vi "WriteData.vi"(6 "TransmissionType":T1, 8 "error in (no error)":errorcluster, 10 "Command":string, 11 "ControlState in":T2 {"ChainMask" format="0x%02x"}) -> (0 "error out":errorcluster, 1 "Data Written?":bool, 2 "return count":u32, 3 "ControlState out":T2 {"ChainMask" format="0x%02x"})   [LabVIEW 2018, in "ArduinoSerialBling.lvlib"]
uses:
  ArduinoSerialBling.lvlib
  ControlState.ctl
  ConnectionType.ctl
  UdpConnection.ctl
  ChainState.ctl
  TransmissionType.ctl
  <vilib>/Instr/_visa.llb/VISA Flush IO Buffer Mask.ctl
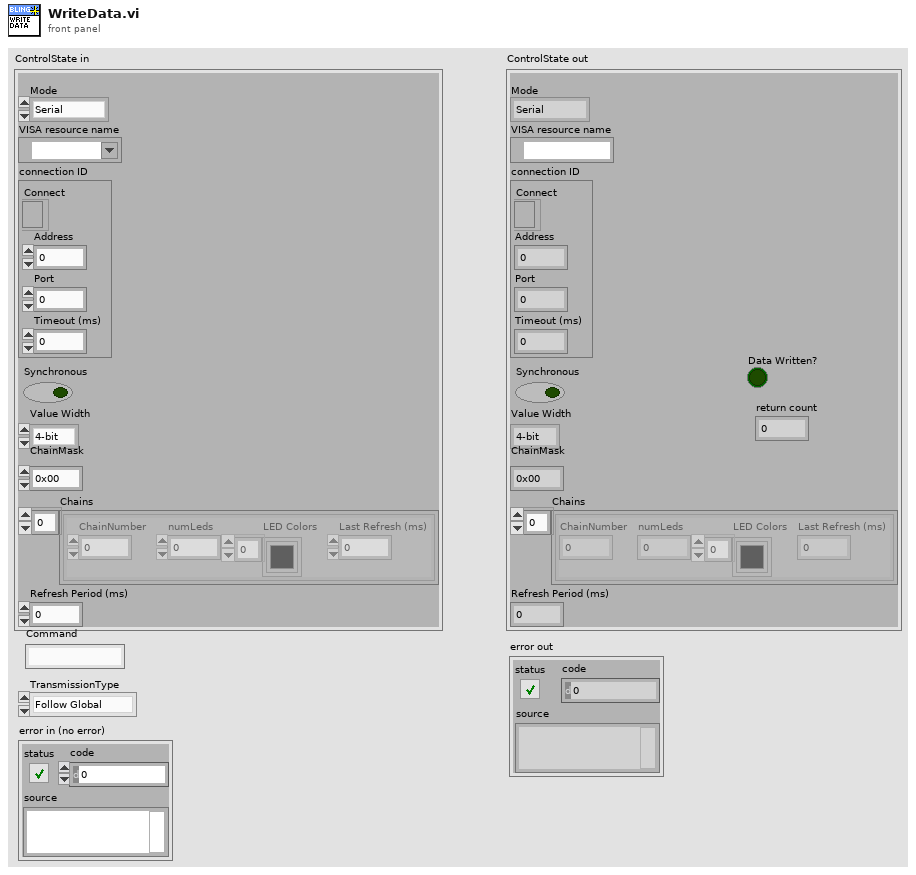
[diagram p1: front panel]
types:
  T1 = typedef "ArduinoSerialBling.lvlib/TransmissionType.ctl" = enum16{"Follow Global", "Asynchronous", "Synchronous"}
  T2 = typedef "ArduinoSerialBling.lvlib/ControlState.ctl" = cluster{"Mode":T3, "VISA resource name":refnum<visa-resource-name>, "connection ID":T4, "Synchronous":bool, "Value Width":enum16{"4-bit", "8-bit"}, "ChainMask":u8, "Chains":T5[], "Refresh Period (ms)":u32}
  T3 = typedef "ConnectionType.ctl" = enum16{"Serial", "Ethernet", "Offline"}
  T4 = typedef "UdpConnection.ctl" = cluster{"Connect":refnum<k16>, "Address":u32, "Port":u16, "Timeout (ms)":i32}
  T5 = typedef "ArduinoSerialBling.lvlib/ChainState.ctl" = cluster{"ChainNumber":u8, "numLeds":u8, "LED Colors":u32[], "Last Refresh (ms)":u32}
  T6 = typedef "VISA Flush IO Buffer Mask.ctl" = u16
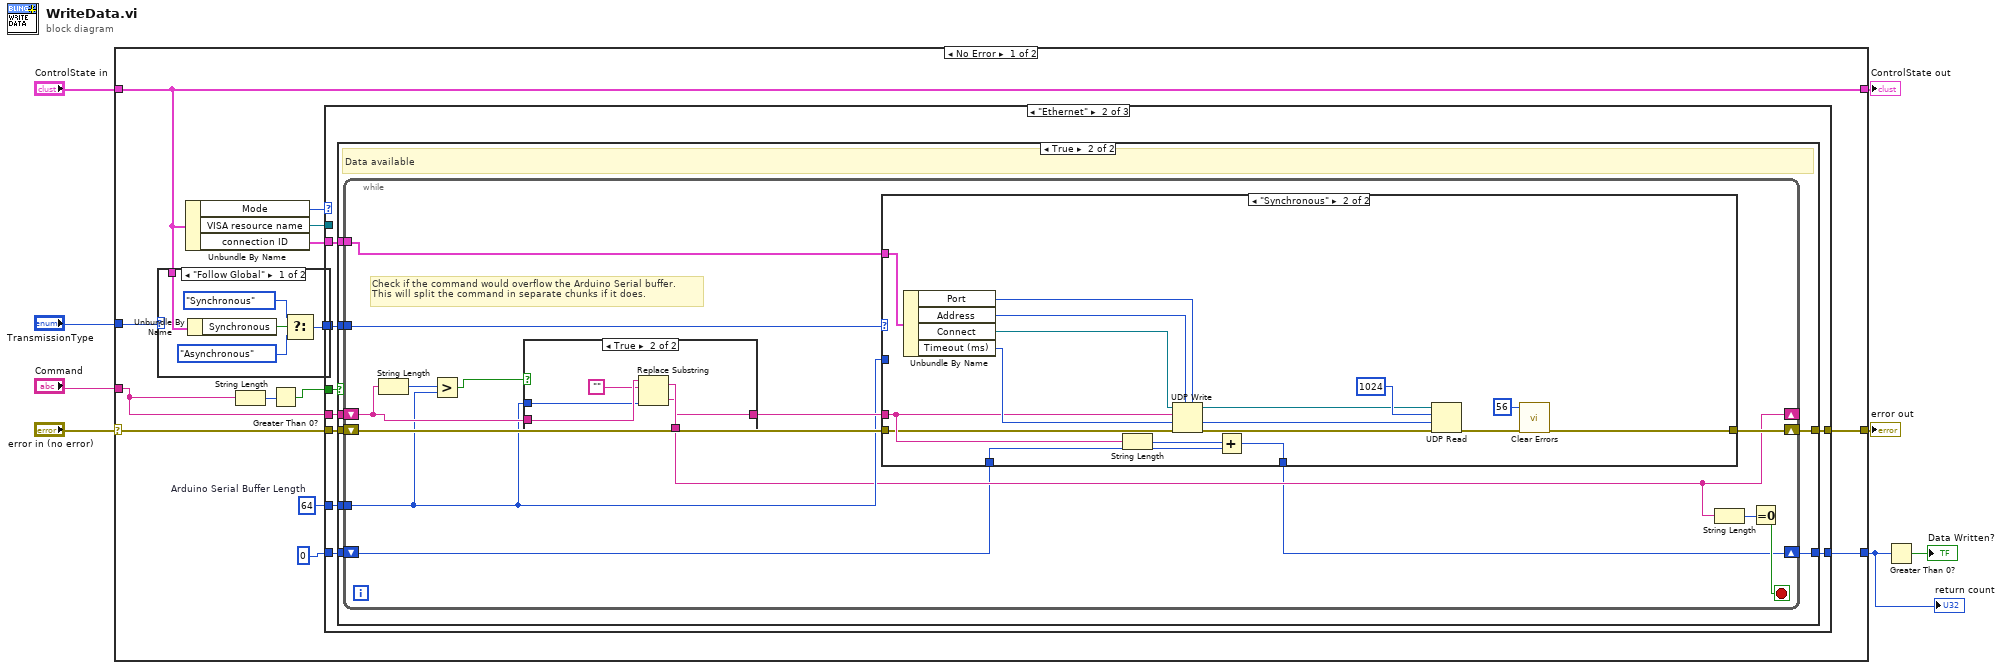
[diagram p0: block diagram]
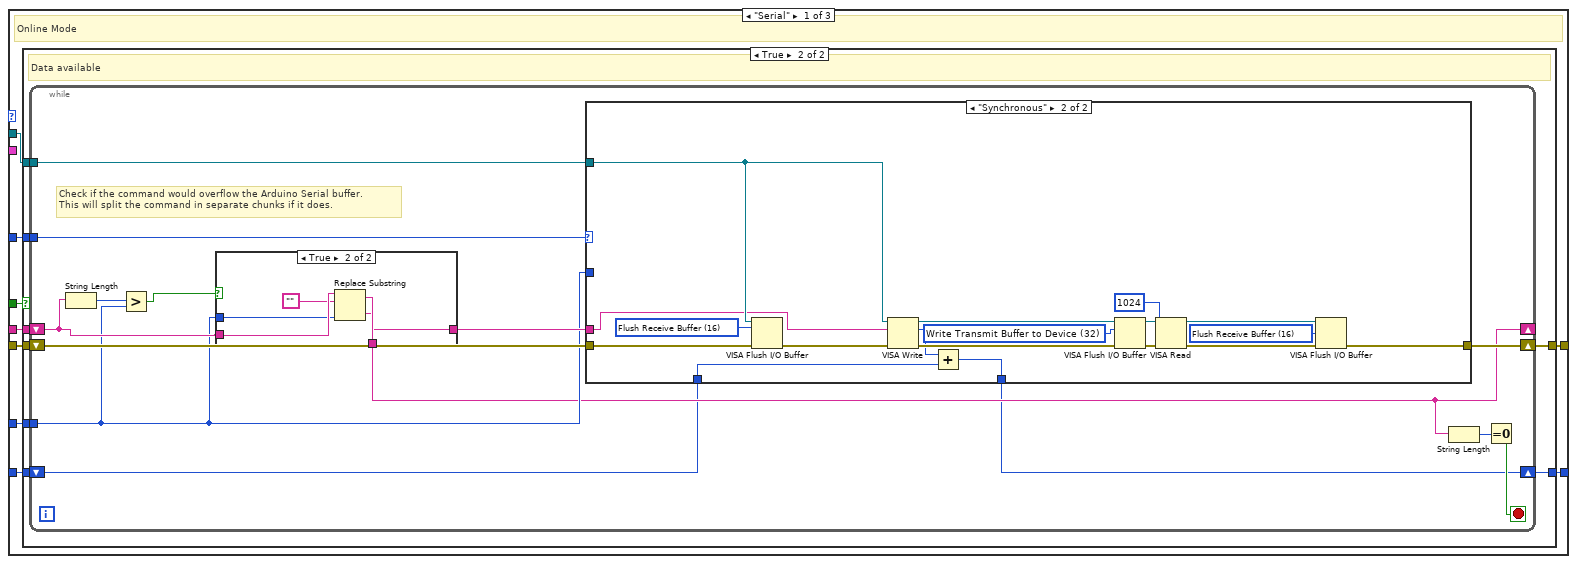
[diagram p2: hidden frame]
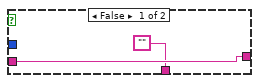
[diagram p4: hidden frame]
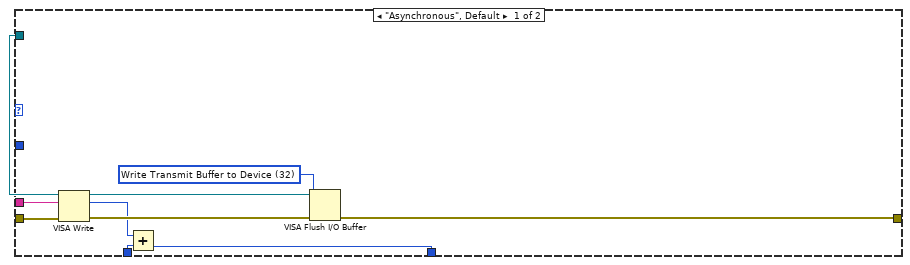
[diagram p5: hidden frame]
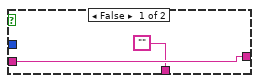
[diagram p7: hidden frame]
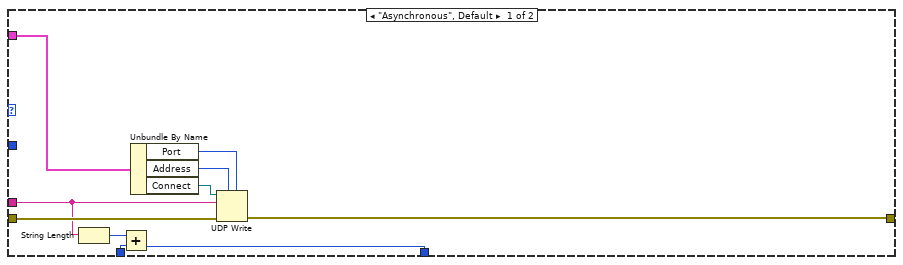
[diagram p8: hidden frame]
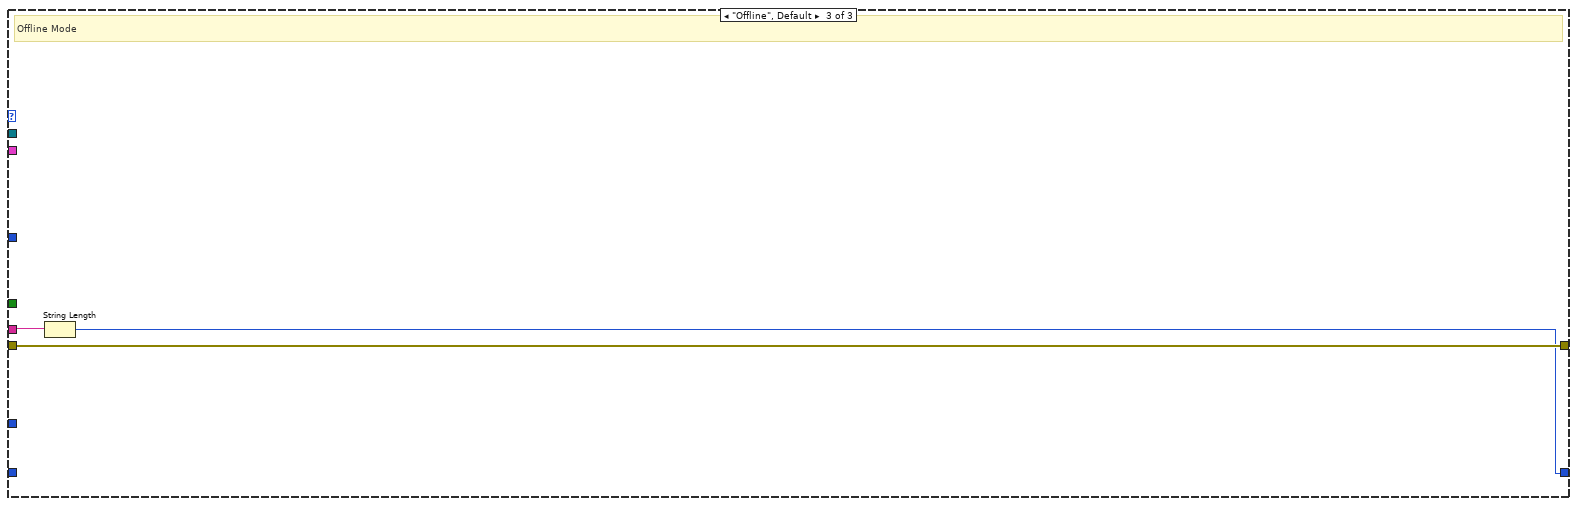
[diagram p9: hidden frame]
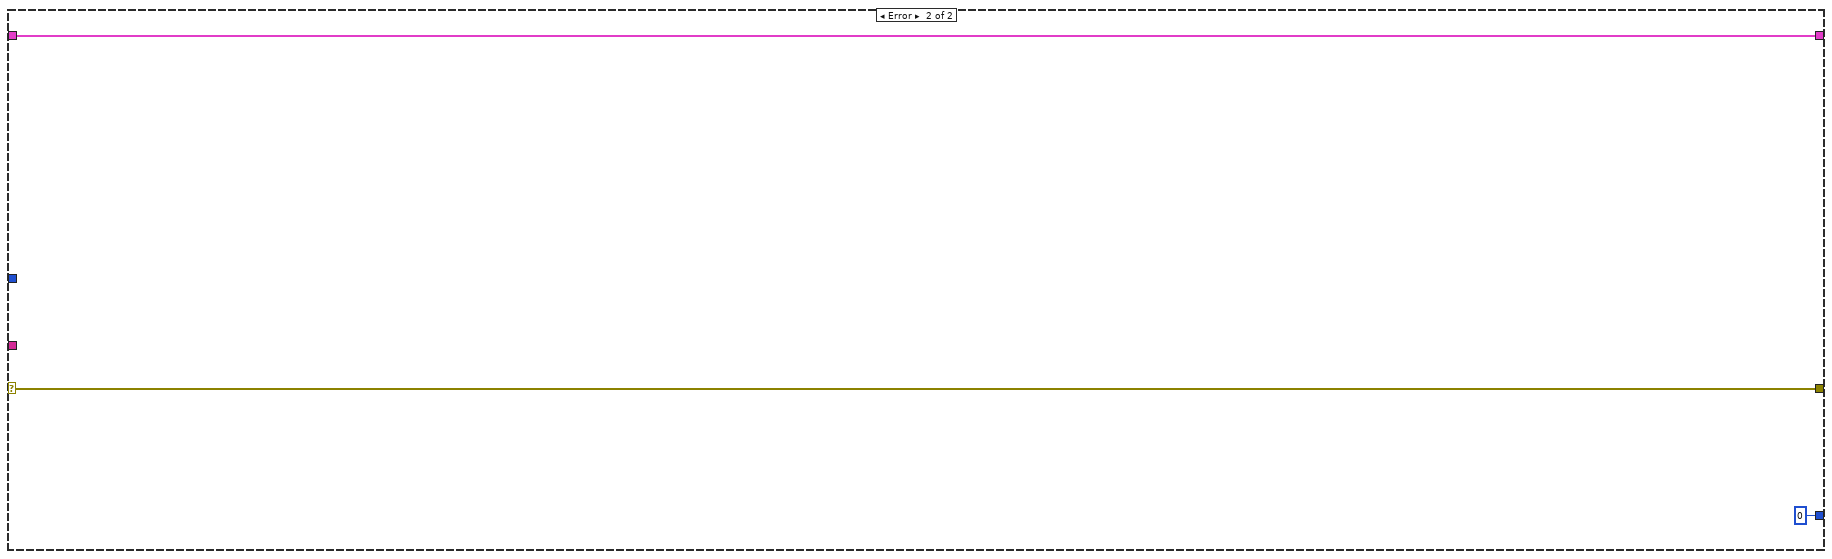
[diagram p11: hidden frame]
diagram:
  n1 = case shown="No Error" "error in (no error)" {
    selector: "error in (no error)" -> [w11 w168]
    tunnel: [w20 w168] -> w7
    tunnel: "ControlState in" -> [w19 w167]
    tunnel: [w19 w167] -> w5
    tunnel: "Command" -> [w10 _]
    tunnel: "TransmissionType" -> [w22 _]
    tunnel: [w13 0] -> w2
    frame No Error {
      w17 = 64  # Arduino Serial Buffer Length
      n2 = case shown="\"Follow Global\"" w22 {
        selector: w22 -> [_ w165]
        tunnel: w19 -> [w164 _]
        tunnel: [w160 w165] -> w21
        frame "Follow Global" {
          n3 = Unbundle By Name(w164) -> ("Synchronous"=w163:bool)
          n4 = Select(t=TransmissionType."Synchronous" ("TransmissionType"), s=w163, f=TransmissionType."Asynchronous") -> (s? t:f=w160:T1)
        }
        frame Default {
        }
      }
      n5 = Unbundle By Name(w19) -> ("Mode"=w12:T3, "VISA resource name"=w18:refnum<visa-resource-name>, "connection ID"=w9:T4)
      n6 = String Length(string=w10) -> (length=w15:i32)
      n7 = Greater Than 0?(x=w15) -> (x > 0?=w14:bool)
      n8 = case shown="\"Ethernet\"" w12 {
        tunnel: w21 -> [w31 w93 _]
        tunnel: w11 -> [w30 w95 w159]
        tunnel: [w29 w99 w159] -> w20
        tunnel: w18 -> [w28 _ _]
        tunnel: w17 -> [w27 w96 _]
        tunnel: 0 -> [w26 w97 _]
        tunnel: w10 -> [w25 w94 w158]
        tunnel: w14 -> [w24 w91 _]
        tunnel: [w23 w98 w157] -> w13
        tunnel: w9 -> [_ w92 _]
        frame "Serial" {
          # "Online Mode"
          n9 = case shown="True" w24 {
            tunnel: w31 -> [_ w41]
            tunnel: w30 -> [w32 w40]
            tunnel: [w32 w39] -> w29
            tunnel: w28 -> [_ w38]
            tunnel: w27 -> [_ w37]
            tunnel: w25 -> [_ w36]
            tunnel: w26 -> [w33 w35]
            tunnel: [w33 w34] -> w23
            frame False {
              # "No data available"
            }
            frame True {
              # "Data available"
              n10 = while {
                tunnel: w41 -> [w55]
                tunnel: w38 -> [w52]
                shift-right: [w53] -> w39
                shift-left: w40 -> [w54]
                shift-right: [w46] -> _
                shift-left: w36 -> [w49]
                tunnel: w37 -> [w47]
                shift-right: [w42] -> w34
                shift-left: w35 -> [w43]
                stop <- w44 stop-if-true
                # "Check if the command would overflow the Arduino Serial buffer.\nThis will split the command in separate chunks if it does."
                n11 = String Length(string=w49) -> (length=w51:i32)
                n12 = Greater?(x=w51, y=w47) -> (0:w50:bool)
                n13 = case shown="True" w50 {
                  tunnel: w49 -> [w57 w62]
                  tunnel: w47 -> [_ w61]
                  tunnel: ["" w59] -> w46
                  tunnel: [w57 w58] -> w48
                  frame False {
                  }
                  frame True {
                    n14 = Replace Substring(2:w61, 4:"", 5:w62) -> (0:w58:string, 1:w59:string)  [unwired: 1 in]
                  }
                }
                n15 = case shown="\"Synchronous\"" w55 {
                  tunnel: w54 -> [w72 w88]
                  tunnel: [w67 w90] -> w53
                  tunnel: w52 -> [w71 w87]
                  tunnel: w48 -> [w66 w76]
                  tunnel: w47 -> [_ _]
                  tunnel: w43 -> [w64 w74]
                  tunnel: [w63 w73] -> w42
                  frame "Asynchronous", Default {
                    w68 = T6 32 items=["Flush Receive Buffer"=16, "Write Transmit Buffer to Device"=32, "Flush Receive Buffer (No I/O)"=64, "Flush Transmit Buffer"=128] ("Mask")
                    n16 = VISA Write(VISA resource name=w71, write buffer=w66, error in (no error)=w72) -> (VISA resource name out=w69:refnum<visa-resource-name>, return count=w65:u32, error out=w70:errorcluster)
                    n17 = Add(x=w65, y=w64) -> (x+y=w63:u32)
                    n18 = VISA Flush I/O Buffer(VISA resource name=w69, mask (16)=w68, error in (no error)=w70) -> (error out=w67:errorcluster)  [unwired: 1 out]
                  }
                  frame "Synchronous" {
                    w79 = T6 16 items=["Flush Receive Buffer"=16, "Write Transmit Buffer to Device"=32, "Flush Receive Buffer (No I/O)"=64, "Flush Transmit Buffer"=128] ("Mask")
                    w80 = T6 32 items=["Flush Receive Buffer"=16, "Write Transmit Buffer to Device"=32, "Flush Receive Buffer (No I/O)"=64, "Flush Transmit Buffer"=128] ("Mask")
                    w86 = T6 16 items=["Flush Receive Buffer"=16, "Write Transmit Buffer to Device"=32, "Flush Receive Buffer (No I/O)"=64, "Flush Transmit Buffer"=128] ("Mask")
                    n19 = VISA Flush I/O Buffer(VISA resource name=w87, mask (16)=w86, error in (no error)=w88) -> (error out=w89:errorcluster)  [unwired: 1 out]
                    n20 = VISA Write(VISA resource name=w87, write buffer=w76, error in (no error)=w89) -> (VISA resource name out=w83:refnum<visa-resource-name>, return count=w75:u32, error out=w82:errorcluster)
                    n21 = Add(x=w75, y=w74) -> (x+y=w73:u32)
                    n22 = VISA Flush I/O Buffer(VISA resource name=w83, mask (16)=w80, error in (no error)=w82) -> (VISA resource name out=w84:refnum<visa-resource-name>, error out=w85:errorcluster)
                    n23 = VISA Read(VISA resource name=w84, byte count=u32 1024, error in (no error)=w85) -> (VISA resource name out=w78:refnum<visa-resource-name>, error out=w77:errorcluster)  [unwired: 2 out]
                    n24 = VISA Flush I/O Buffer(VISA resource name=w78, mask (16)=w79, error in (no error)=w77) -> (error out=w90:errorcluster)  [unwired: 1 out]
                  }
                }
                n25 = String Length(string=w46) -> (length=w45:i32)
                n26 = Equal To 0?(x=w45) -> (x = 0?=w44:bool)
              }
            }
          }
        }
        frame "Ethernet" {
          n27 = case shown="True" w91 {
            tunnel: w93 -> [_ w109]
            tunnel: w95 -> [w100 w108]
            tunnel: [w100 w107] -> w99
            tunnel: w96 -> [_ w106]
            tunnel: w94 -> [_ w105]
            tunnel: w97 -> [w101 w104]
            tunnel: [w101 w103] -> w98
            tunnel: w92 -> [_ w102]
            frame False {
              # "No data available"
            }
            frame True {
              # "Data available"
              n28 = while {
                tunnel: w109 -> [w123]
                shift-right: [w121] -> w107
                shift-left: w108 -> [w122]
                shift-right: [w115] -> _
                shift-left: w105 -> [w118]
                tunnel: w106 -> [w116]
                shift-right: [w111] -> w103
                shift-left: w104 -> [w112]
                tunnel: w102 -> [w110]
                stop <- w113 stop-if-true
                # "Check if the command would overflow the Arduino Serial buffer.\nThis will split the command in separate chunks if it does."
                n29 = String Length(string=w118) -> (length=w120:i32)
                n30 = Greater?(x=w120, y=w116) -> (0:w119:bool)
                n31 = case shown="True" w119 {
                  tunnel: w118 -> [w125 w130]
                  tunnel: w116 -> [_ w129]
                  tunnel: ["" w127] -> w115
                  tunnel: [w125 w126] -> w117
                  frame False {
                  }
                  frame True {
                    n32 = Replace Substring(2:w129, 4:"", 5:w130) -> (0:w126:string, 1:w127:string)  [unwired: 1 in]
                  }
                }
                n33 = case shown="\"Synchronous\"" w123 {
                  tunnel: w122 -> [w140 w143]
                  tunnel: [w137 w142] -> w121
                  tunnel: w110 -> [w136 w153]
                  tunnel: w117 -> [w131 w144]
                  tunnel: w116 -> [_ _]
                  tunnel: w112 -> [w139 w155]
                  tunnel: [w138 w154] -> w111
                  frame "Asynchronous", Default {
                    n34 = String Length(string=w131) -> (length=w132:i32)
                    n35 = Add(x=w132, y=w139) -> (x+y=w138:i32)
                    n36 = Unbundle By Name(w136) -> ("Port"=w134:u16, "Address"=w135:u32, "Connect"=w133:refnum<k16>)
                    n37 = UDP Write(address=w135, port or service name=w134, connection ID=w133, data in=w131, 8:w140) -> (error out=w137:errorcluster)  [unwired: 1 in, 1 out]
                  }
                  frame "Synchronous" {
                    n38 = Unbundle By Name(w153) -> ("Port"=w151:u16, "Address"=w150:u32, "Connect"=w152:refnum<k16>, "Timeout (ms)"=w147:i32)
                    n39 = String Length(string=w144) -> (length=w145:i32)
                    n40 = UDP Write(address=w150, port or service name=w151, connection ID=w152, data in=w144, 8:w143, 9:w147) -> (error out=w149:errorcluster, 3:w146:refnum<k16>)
                    n41 = Add(x=w145, y=w155) -> (x+y=w154:i32)
                    n42 = UDP Read(connection ID=w146, max size (548)=u32 1024 ("byte count"), timeout ms (25000)=w147, 8:w149) -> (error out=w148:errorcluster)  [unwired: 4 out]
                    n43 = call <vilib>:"Clear Errors.vi"("error in (no error)"=w148, "specific error code to clear (0: all)"=56) -> ("error out"=w142:errorcluster)  [unwired: 4 in, 1 out]
                  }
                }
                n44 = String Length(string=w115) -> (length=w114:i32)
                n45 = Equal To 0?(x=w114) -> (x = 0?=w113:bool)
              }
            }
          }
        }
        frame "Offline", Default {
          # "Offline Mode"
          n46 = String Length(string=w158) -> (length=w157:i32)
        }
      }
    }
    frame Error {
    }
  }
  "ControlState out" <- w5
  "error out" <- w7
  "return count" <- w2
  n47 = Greater Than 0?(x=w2) -> (x > 0?=→"Data Written?":bool)
